vi "Power_DUT.vi"(8 "error in (no error)":errorcluster, 10 "Parameters":string, 11 "reference in":refnum<class "Test_NanoP5.lvclass">) -> (0 "error out":errorcluster, 2 "Result":bool, 3 "reference out":refnum<class "Test_NanoP5.lvclass">)   [LabVIEW 2019]
uses:
  Test_NanoP5.lvclass
  <vilib>/addons/_JKI.lib/Serialization/JSON/JKI JSON Serialization.lvlib
  Components/SwitchBase.lvlibp/SwitchBase.lvclass
  ParameterTypes/PowerDUT.ctl
panel:
  in  "Parameter_Type":T1
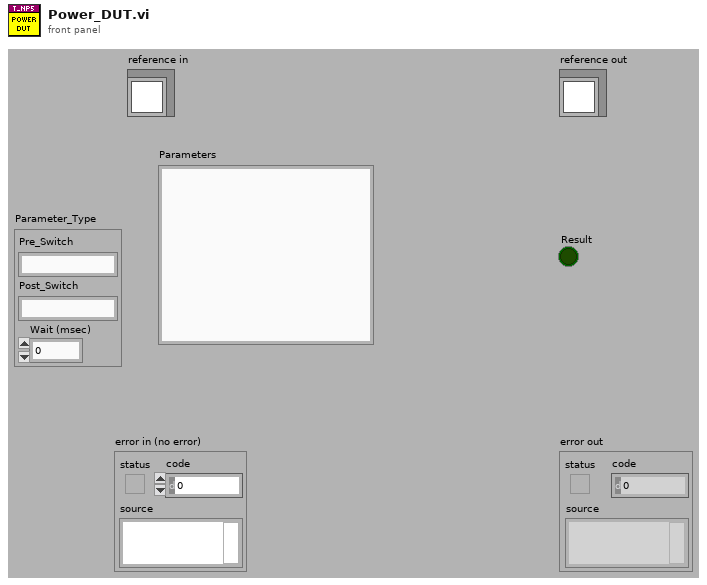
[diagram p1: front panel]
types:
  T1 = typedef "Test_NanoP5.lvlib/Test_NanoP5.lvclass/PowerDUT.ctl" = cluster{"Pre_Switch":string, "Post_Switch":string, "Wait (msec)":u32}
  T2 = typedef "Test_NanoP5.lvlib/Test_NanoP5.lvclass/ObjectAttributes.ctl" = cluster{"Config":T3, "DMM":refnum<class "DMM_Keysight_34980A.lvclass">, "LCR":refnum<class "LCR_BK891.lvclass">, "PSU":refnum<class "PSU_Base.lvclass">, "Switch_Manager":refnum<class "SwitchBase.lvclass">, "Switch_Motor":refnum<class "SwitchBase.lvclass">, "NanoP5":refnum<class "NanoP5.lvclass">}
  T3 = typedef "Test_NanoP5.lvlib/Test_NanoP5.lvclass/Config.ctl" = cluster{"default":string}
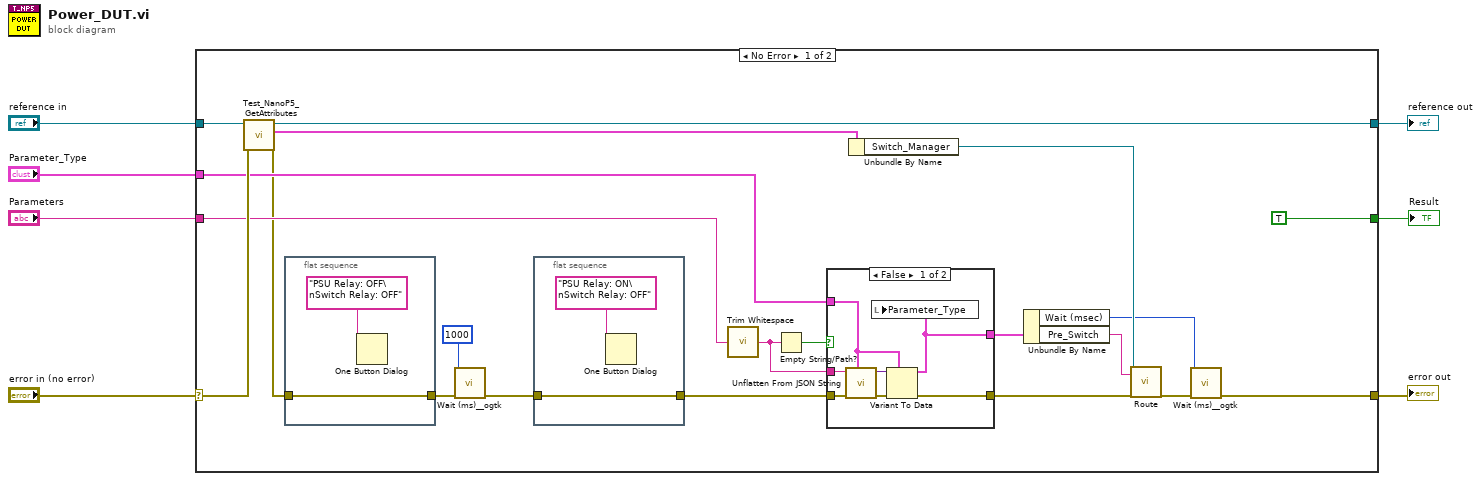
[diagram p0: block diagram]
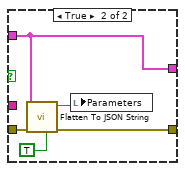
[diagram p2: hidden frame]
diagram:
  n1 = case shown="No Error" "error in (no error)" {
    selector: "error in (no error)" -> [w28 w46]
    tunnel: [w14 w46] -> w6
    tunnel: [w26 w45] -> w4
    tunnel: "reference in" -> [w27 w45]
    tunnel: "Parameters" -> [w19 _]
    tunnel: "Parameter_Type" -> [w20 _]
    tunnel: [TRUE _] -> w1
    frame No Error {
      n2 = call "Test_NanoP5_GetAttributes.vi"("error in (no error)"=w28, "reference in"=w27) -> ("error out"=w12:errorcluster, "Data"=w25:T2, "reference out"=w26:refnum<class "Test_NanoP5.lvclass">)  [unwired: 6 in, 1 out]
      n3 = flat-sequence {
        tunnel: w12 -> [w32]
        tunnel: [w32] -> w11
        frame #0 {
          n4 = One Button Dialog(message="PSU Relay: OFF\nSwitch Relay: OFF") -> ()  [unwired: 1 in, 1 out]
        }
      }
      n5 = call <userlib>:"Wait (ms)__ogtk.vi"("error in (no error)"=w11, "milliseconds to wait"=u32 1000) -> ("error out"=w9:errorcluster)  [unwired: 8 in, 1 out]
      n6 = flat-sequence {
        tunnel: w9 -> [w30]
        tunnel: [w30] -> w8
        frame #0 {
          n7 = One Button Dialog(message="PSU Relay: ON\nSwitch Relay: OFF") -> ()  [unwired: 1 in, 1 out]
        }
      }
      n8 = call <vilib>:"Trim Whitespace.vi"("string"=w19) -> ("trimmed string"=w22:string)  [unwired: 1 in]
      n9 = Empty String/Path?(string/path=w22) -> (empty?=w21:bool)
      n10 = case shown="False" w21 {
        tunnel: w8 -> [w37 w43]
        tunnel: w20 -> [w36 w42]
        tunnel: [w35 w44] -> w15
        tunnel: [w33 w42] -> w18
        tunnel: w22 -> [w34 _]
        frame False {
          n11 = call <vilib>:"Unflatten From JSON String.vi"("Type and Defaults"=w36, "error in (no error)"=w37, "JSON String"=w34) -> ("error out"=w39:errorcluster, "Variant"=w38:variant)  [unwired: 7 in]
          n12 = Variant To Data(error in=w39, type=w36, Variant=w38) -> (data=w33:T1, error out=w35:errorcluster)
          n13 = local write "Parameter_Type"(w33) -> ()
        }
        frame True {
          n14 = call <vilib>:"Flatten To JSON String.vi"("Enums As String (F)"=TRUE, "error in (no error)"=w43, "Variant"=w42) -> ("error out"=w44:errorcluster, "JSON String"=w41:string)  [unwired: 7 in]
          n15 = local write "Parameters"(w41) -> ()
        }
      }
      n16 = Unbundle By Name(w25) -> ("Switch_Manager"=w24:refnum<class "SwitchBase.lvclass">)
      n17 = Unbundle By Name(w18) -> ("Wait (msec)"=w16:u32, "Pre_Switch"=w17:string)
      n18 = call-dynamic "Route.vi"("reference in"=w24, "channel 1"=w17, "error in (no error)"=w15) -> ("error out"=w23:errorcluster)  [unwired: 15 in, 1 out]
      n19 = call <userlib>:"Wait (ms)__ogtk.vi"("error in (no error)"=w23, "milliseconds to wait"=w16) -> ("error out"=w14:errorcluster)  [unwired: 8 in, 1 out]
    }
    frame Error {
    }
  }
  "Result" <- w1
  "error out" <- w6
  "reference out" <- w4
